vi "COD测量模式全局.vi"() -> ()   [LabVIEW 2016, in "斯坦道CODMn.lvlib"]
panel:
  out "测量模式":string
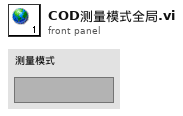
[diagram p1: front panel]
diagram:
